vi "Jog Multiple Steps.vi"(8 "error in (no error)":errorcluster, 9 "StepAmount":dbl, 10 "Jog Direction":T1, 11 "Thorlabs in":refnum<class "Thorlabs.lvclass">) -> (0 "error out":errorcluster, 3 "Thorlabs out":refnum<class "Thorlabs.lvclass">)   [LabVIEW 2018, in "Thorlabs.lvlib" / "Thorlabs.lvclass"]
doc: "Commands the Axis to jog the specified direction in a multiple single step sizes."
uses:
  Thorlabs.lvclass
  PPLs/Axis/Parent/Axis.lvlibp/Custom Controls/Jog Direction.ctl
  PPLs/Axis/Parent/Axis.lvlibp
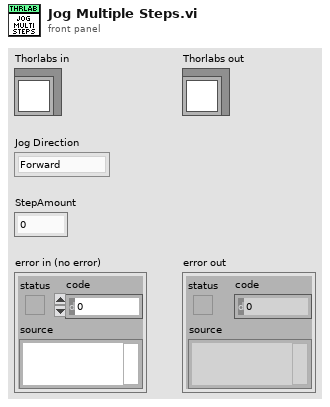
[diagram p1: front panel]
types:
  T1 = typedef "Axis.lvlibp/Jog Direction.ctl" = enum16{"Forward", "Backward"}
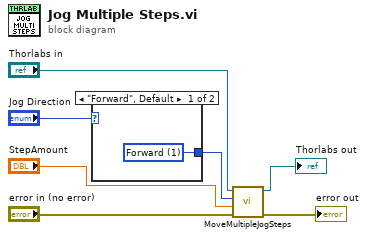
[diagram p0: block diagram]
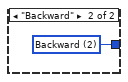
[diagram p2: hidden frame]
diagram:
  n1 = case shown="\"Forward\", Default" "Jog Direction" {
    tunnel: [w8 w9] -> w4
    frame "Forward", Default {
      w8 = 1 items=["Forward"=1, "Backward"=2] ("direction")
    }
    frame "Backward" {
      w9 = 2 items=["Forward"=1, "Backward"=2] ("direction")
    }
  }
  n2 = call "MoveMultipleJogSteps.vi"("Error In"="error in (no error)", "Step Amounts"="StepAmount", "direction"=w4, "Thorlabs In"="Thorlabs in") -> ("Error Out"=→"error out":errorcluster, "Thorlabs Out"=→"Thorlabs out":refnum<class "Thorlabs.lvclass">)  [unwired: 6 in]
